vi "Teleop.vi"(10 "Match Info":T1={"Autonomous Elapsed Seconds"=0.0, "TeleOp Elapsed Seconds"=0.0, "Disabled Elapsed Seconds"=0.0, "Visited Autonomous"=FALSE, "Visited TeleOp"=FALSE, "Visited Disabled"=FALSE, "Autonomous Settings"={"Autonomous Style"=enum."Independent", "VI Refnum"=refnum}}, 11 "Call Context":T2) -> ()   [LabVIEW 2016]
doc: "This VI is called for each TeleOp packet received from the DS where the robot is not disabled. It is often used to read from the joysticks and update I/O or to update setpoints for timed control loops. It should complete and return within 20 milliseconds or it may miss DS packets."
uses:
  <vilib>/Rock Robotics/WPI/DriverStation/WPI_DriverStationDerivedRobotMode.ctl
  <vilib>/Rock Robotics/WPI/DriverStation/WPI_DriverStationMatch Info.ctl
  <vilib>/Rock Robotics/WPI/Solenoid/WPI_SolenoidValue.ctl
  <vilib>/Rock Robotics/WPI/ThirdParty/CanMotor/TalonSRX/WPI_CANTalonSRX_APIControlMode.ctl
  <vilib>/Rock Robotics/WPI/Utilities/WPI_GetSetVariantRefNum.vi
  <vilib>/Rock Robotics/Network Tables/NT Write Boolean Array.vi
  <vilib>/Rock Robotics/Network Tables/NT Write Numeric Array.vi
  <vilib>/Rock Robotics/Network Tables/NT Write Boolean.vi
  <vilib>/Rock Robotics/WPI/Solenoid/WPI_SolenoidSetEnum.vi
panel:
  out "Applied Throttle":dbl
  in  "Max Velocity":i32=63320
  in  "F":dbl
  in  "Speed PID":bool
  out "Setpoint vs Velocity":cluster{dbl, "Sensor Velocity":dbl}(graph)
  in  "Setpoint Control":bool
  out "Closed Loop Error":dbl(graph)
  in  "Setpoint (RPM)":dbl
  in  "D":dbl
  in  "I":dbl
  in  "P":dbl
  in  "Apply":bool
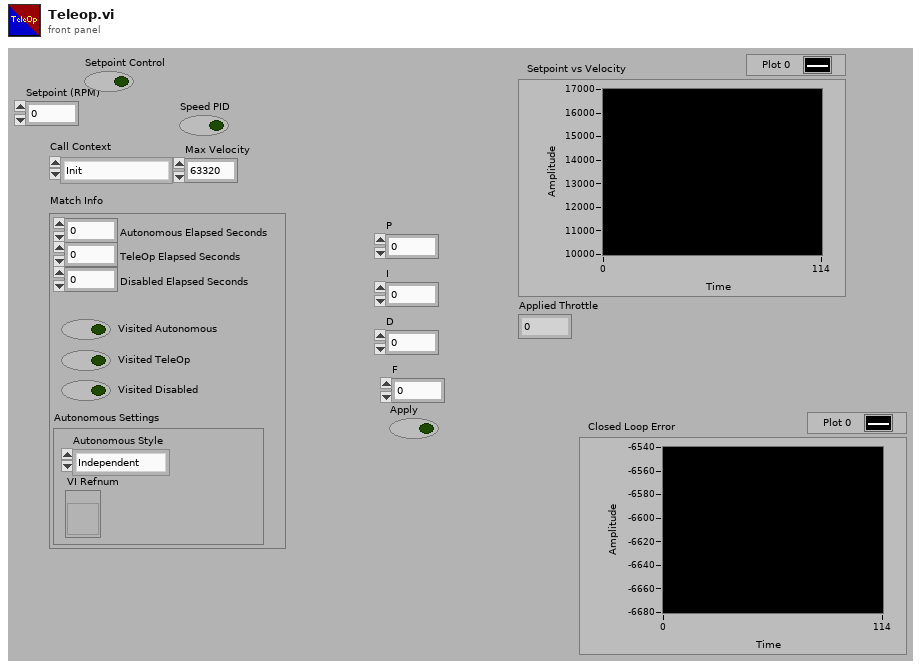
[diagram p1: front panel]
types:
  T1 = typedef "WPI_DriverStationMatch Info.ctl" = cluster{"Autonomous Elapsed Seconds":dbl, "TeleOp Elapsed Seconds":dbl, "Disabled Elapsed Seconds":dbl, "Visited Autonomous":bool, "Visited TeleOp":bool, "Visited Disabled":bool, "Autonomous Settings":cluster{"Autonomous Style":enum16{"Iterative", "Independent"}, "VI Refnum":refnum<vi>}}
  T2 = typedef "WPI_DriverStationDerivedRobotMode.ctl" = enum16{"Init", "Execute", "Stop"}
  T3 = typedef "WPI_JoystickDevRef.ctl" = cluster{"Device":T4}
  T4 = typedef "WPI_JoystickDeviceEnum.ctl" = enum16{"USB 0", "USB 1", "USB 2", "USB 3", "USB 4", "USB 5"}
  T5 = typedef "WPI_CANTalonSRX_APIControlMode.ctl" = enum8{"Percent VBus", "Speed", "Position", "Slave", "Unchanged / Invalid", "Voltage Compensation", "Current", "Motion Profile", "Motion Magic"}
  T6 = typedef "WPI_RobotDriveDevRef.ctl" = cluster{"DevStatus":errorcluster, "Motors[]":T7[], "Square Inputs":bool, "Max Output":dbl}
  T7 = typedef "WPI_MotorControlDeviceRef.ctl" = cluster{"DeviceStatus":errorcluster, "Type":T8, "PWM":cluster{"PWM Channel":T9, "DeadBand":T10}, "CAN":cluster{"Device Number":u8, "SetOutput VI Ref":variant, "GetOutput VI Ref":variant, "Enable VI Ref":variant, "Disable VI Ref":variant, "Data":variant}, "Invert":bool}
  T8 = typedef "WPI_MotorControlType.ctl" = enum16{"PWM", "CAN"}
  T9 = typedef "FPGA_DIOPWMChannel.ctl" = enum8{"PWM 0", "PWM 1", "PWM 2", "PWM 3", "PWM 4", "PWM 5", "PWM 6", "PWM 7", "PWM 8", "PWM 9", "PWM MXP 0", "PWM MXP 1", "PWM MXP 2", "PWM MXP 3", "PWM MXP 4", "PWM MXP 5", "PWM MXP 6", "PWM MXP 7", "PWM MXP 8", "PWM MXP 9", "Invalid"}
  T10 = typedef "WPI_PWMDeadband.ctl" = cluster{"Name":string, "maxPositivePwm":i32, "minPositivePwm":i32, "centerPwm":i32, "maxNegativePwm":i32, "minNegativePwm":i32, "angularRange":u16}
  T11 = typedef "WPI_CANTalonSRX_GlobalStatus.ctl" = cluster{"Applied Throttle":dbl, "Module Enabled":bool, "CAN Error":errorcluster, "Closed Loop Error":dbl, "Forward Limit Switch Closed":bool, "Reverse Limit Switch Closed":bool, "Sensor Position":dbl, "Sensor Velocity":dbl, "Current":dbl, "Sticky Fault - Over Temp":bool, "Sticky Fault - Under Voltage":bool, "Sticky Fault - Forward Limit":bool, "Sticky Fault - Reverse Limit":bool, "Sticky Fault - Forward Soft Limit":bool, "Sticky Fault - Reverse Soft Limit":bool, "Brake is Enabled":bool, "Encoder Position":dbl, "Encoder Velocity":dbl, "Encoder Index Count":dbl, "Encoder A Pin State":bool, "Encoder B Pin State":bool, "Encoder Index Pin State":bool, "Analog In":dbl, "Analog In Velocity":dbl, "Temperature (C)":dbl, "Battery Voltage":dbl, "Control 5 Is Supported":bool, "Current Profile Slot Select":dbl, "Pos Div 8":bool, "Vel Div 4":bool, "Pulse Width Position":i32, "Pulse Width Velocity":i32, "Pulse Width Rise To Rise (us)":i32, "Pulse Width Rise To Fall (us)":i32, "Mot Prof Active Is Under Run":bool, "Mot Prof Active Has Under Run":bool, "Mot Prof Active Is Last":bool, "Mot Prof Active Velocity Only":bool, "Mot Prof Active Is Valid":bool, "Mot Prof Buffer Is Full":bool, "Mot Prof Active Profile Slot Select":i32, "Mot Prof NextID":i32, "Mot Prof Count":i32, "Mot Prof Active Velocity":dbl, "Mot Prof Active Position":dbl, "Mot Prof Output Enable":i32}
  T12 = typedef "WPI_SolenoidValue.ctl" = enum16{"Off", "On", "Forward", "Reverse"}
  T13 = typedef "WPI_SolenoidDevRef.ctl" = cluster{"DevStatus":errorcluster, "Pneumatics Control Module":u8, "Forward Solenoid Channel":T14, "Reverse Solenoid Channel":T14}
  T14 = typedef "WPI_SolenoidChannel.ctl" = enum8{"Solenoid 0", "Solenoid 1", "Solenoid 2", "Solenoid 3", "Solenoid 4", "Solenoid 5", "Solenoid 6", "Solenoid 7", "Invalid"}
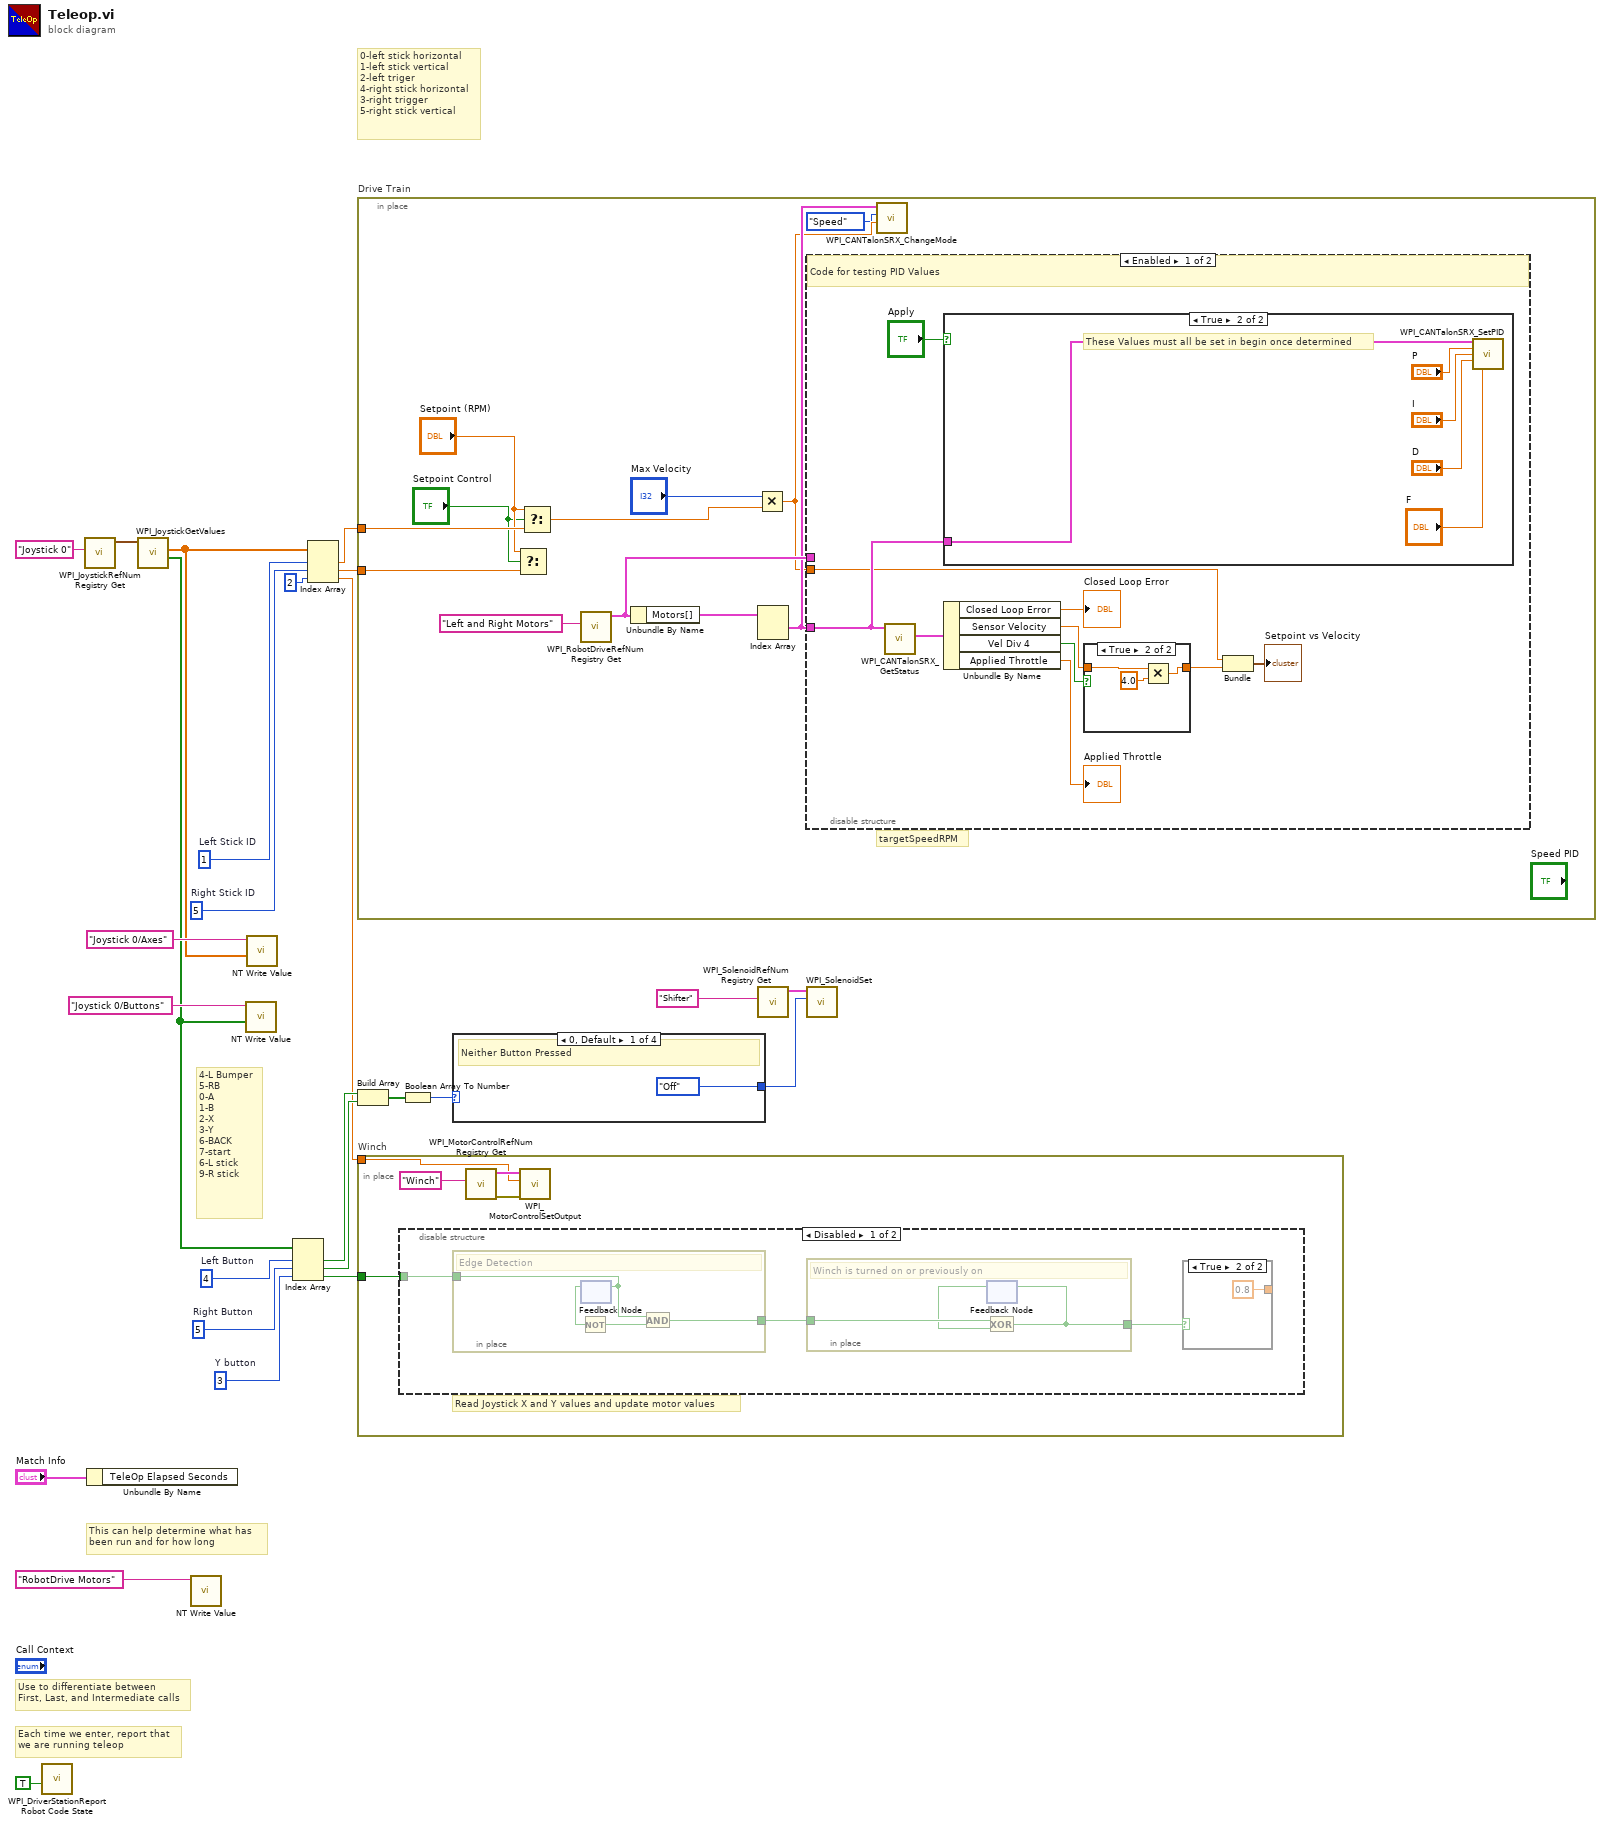
[diagram p0: block diagram]
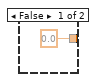
[diagram p5: hidden frame]
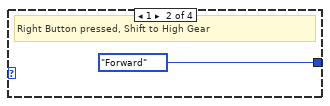
[diagram p7: hidden frame]
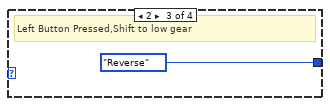
[diagram p8: hidden frame]
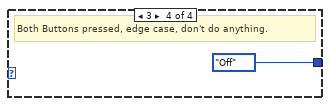
[diagram p9: hidden frame]
diagram:
  w4 = 3  # Y button
  w8 = 1  # Left Stick ID
  w7 = 5  # Right Stick ID
  w9 = 5  # Right Button
  w10 = 4  # Left Button
  # "0-left stick horizontal\n1-left stick vertical\n2-left triger\n4-right stick horizontal\n3-right trigger\n5-right stick vertical"
  # "4-L Bumper\n5-RB\n0-A\n1-B\n2-X\n3-Y\n6-BACK\n7-start\n6-L stick\n9-R stick"
  # "Each time we enter, report that\nwe are running teleop"
  # "Use to differentiate between\nFirst, Last, and Intermediate calls"
  # "This can help determine what has\nbeen run and for how long"
  n1 = call <vilib>:"WPI_DriverStationReport Robot Code State.vi"("TeleOp"=TRUE ("Autonomous")) -> ()  [unwired: 10 in, 1 out]
  n2 = call <vilib>:"WPI_JoystickRefNum Registry Get.vi"("refnum name"="Joystick 0") -> ("JoystickDevRef"=w24:T3)  [unwired: 1 in, 9 out]
  n3 = Unbundle By Name("Match Info") -> ()  [unwired: 1 out]
  n4 = call <vilib>:"WPI_JoystickGetValues.vi"("JoystickDevRef"=w24) -> ("Buttons"=w16:bool[], "Axes"=w20:dbl[])  [unwired: 6 in, 3 out]
  n5 = call-poly <vilib>:"NT Write Value.vi"("Name"="RobotDrive Motors") -> ()  [unwired: 10 in, 1 out]
  n6 = call-poly <vilib>:"NT Write Value.vi"("Boolean Array"=w16, "Name"="Joystick 0/Buttons") -> ()  [unwired: 9 in, 1 out]
  n7 = call-poly <vilib>:"NT Write Value.vi"("Numeric Array"=w20, "Name"="Joystick 0/Axes") -> ()  [unwired: 9 in, 1 out]
  n8 = Index Array(array=w16, index #1=w10, index #2=w9, index #3=w4) -> (element #1=w15:bool, element #2=w14:bool, element #3=w3:bool)
  n9 = Index Array(array=w20, index #1=w8, index #2=w7, index #3=2 ("index")) -> (element #1=w5:dbl, element #2=w6:dbl, element #3=w1:dbl)
  n10 = in-place "Drive Train" {
    in-place-border: w6 -> [w35]
    in-place-border: w5 -> [w37]
    # "targetSpeedRPM"
    n11 = Select(t="Setpoint (RPM)", s="Setpoint Control", f=w35) -> ()  [unwired: 1 out]
    n12 = Select(t="Setpoint (RPM)", s="Setpoint Control", f=w37) -> (s? t:f=w30:dbl)
    n13 = call <vilib>:"WPI_RobotDriveRefNum Registry Get.vi"("refnum name"="Left and Right Motors") -> ("RobotDriveDevRef"=w32:T6)  [unwired: 1 in, 9 out]
    n14 = Unbundle By Name(w32) -> ("Motors[]"=w33:T7[])
    n15 = Multiply(x="Max Velocity", y=w30) -> (x*y=w28:dbl)
    n16 = Index Array(array=w33) -> (element #1=w31:T7)  [unwired: 2 in, 1 out]
    n17 = disable-structure shown="Enabled" {
      disable-tunnel: w32 -> [_ _]
      disable-tunnel: w31 -> [w41 _]
      disable-tunnel: w28 -> [w40 _]
      frame Enabled {
        # "Code for testing PID Values"
        n18 = call <vilib>:"WPI_CANTalonSRX_GetStatus.vi"("CAN Talon SRX Ref"=w41) -> ("Talon SRX Status"=w48:T11)  [unwired: 8 in, 2 out]
        n19 = case shown="True" "Apply" {
          tunnel: w41 -> [_ w53]
          frame False {
          }
          frame True {
            # "These Values must all be set in begin once determined"
            n20 = call <vilib>:"WPI_CANTalonSRX_SetPID.vi"("CAN Talon SRX Ref"=w53, "P"="P", "I"="I", "D"="D", "F"="F") -> ()  [unwired: 9 in, 2 out]
          }
        }
        n21 = Unbundle By Name(w48) -> ("Closed Loop Error"=→"Closed Loop Error":dbl, "Sensor Velocity"=w42:dbl, "Vel Div 4"=w44:bool, "Applied Throttle"=→"Applied Throttle":dbl)
        n22 = case shown="True" w44 {
          tunnel: [w49 w52] -> w43
          tunnel: w42 -> [w49 w51]
          frame False {
          }
          frame True {
            n23 = Multiply(x=w51, y=4.0) -> (x*y=w52:dbl)
          }
        }
        n24 = Bundle(w40, "Sensor Velocity"=w43) -> (→"Setpoint vs Velocity":cluster{dbl, "Sensor Velocity":dbl})  [unwired: 1 in]
      }
      frame Disabled {
      }
    }
    n25 = call <vilib>:"WPI_CANTalonSRX_ChangeMode.vi"("Output"=w28, "Control Mode"=WPI_CANTalonSRX_APIControlMode."Speed", "CAN Talon SRX Ref"=w31) -> ()  [unwired: 7 in, 2 out]
  }
  n26 = Build Array(w15, w14) -> (w13:bool[])
  n27 = in-place "Winch" {
    in-place-border: w3 -> [w59]
    in-place-border: w1 -> [w58]
    # "Read Joystick X and Y values and update motor values"
    n28 = disable-structure shown="Disabled" {
      disable-tunnel: w59 -> [w65 _]
      frame Disabled {
        n29 = in-place {
          in-place-border: w65 -> [w74]
          in-place-border: [w71] -> w64
          # "Edge Detection"
          n30 = feedback #1() -> (w72:bool)  [unwired: 1 in]
          n31 = Not(x=w72) -> (.not. x?=w73:bool)
          n32 = feedback-in #1(w74) -> ()
          n33 = And(x=w74, y=w73) -> (x .and. y?=w71:bool)
        }
        n34 = in-place {
          in-place-border: w64 -> [w68]
          in-place-border: [w67] -> w63
          # "Winch is turned on or previously on"
          n35 = feedback #2() -> (w66:bool)  [unwired: 1 in]
          n36 = Exclusive Or(1:w66, 2:w68) -> (0:w67:bool)
          n37 = feedback-in #2(w67) -> ()
        }
        n38 = case shown="True" w63 {
          tunnel: [0.0 ("Output") 0.8 ("Output")] -> _
          frame False {
          }
          frame True {
          }
        }
      }
      frame Enabled {
      }
    }
    n39 = call <vilib>:"WPI_MotorControlRefNum Registry Get.vi"("refnum name"="Winch") -> ("error out"=w61:errorcluster, "MotorControlDevRef"=w60:T7)  [unwired: 9 in]
    n40 = call <vilib>:"WPI_MotorControlSetOutput.vi"("error in (no error)"=w61, "Output"=w58, "MotorControlDevRef"=w60) -> ()  [unwired: 6 in, 3 out]
  }
  n41 = Boolean Array To Number(Boolean array=w13) -> (number=w12:u32)
  n42 = case shown="0, Default" w12 {
    tunnel: [WPI_SolenoidValue."Off" ("Value") WPI_SolenoidValue."Forward" ("Value") WPI_SolenoidValue."Reverse" ("Value") WPI_SolenoidValue."Off" ("Value")] -> w11
    frame 0, Default {
      # "Neither Button Pressed"
    }
    frame 1 {
      # "Right Button pressed, Shift to High Gear"
    }
    frame 2 {
      # "Left Button Pressed,Shift to low gear"
    }
    frame 3 {
      # "Both Buttons pressed, edge case, don't do anything."
    }
  }
  n43 = call <vilib>:"WPI_SolenoidRefNum Registry Get.vi"("refnum name"="Shifter") -> ("SolenoidDevRef"=w17:T13)  [unwired: 9 in, 1 out]
  n44 = call-poly <vilib>:"WPI_SolenoidSet.vi"("Value"=w11, "SolenoidDevRef"=w17) -> ()  [unwired: 8 in, 2 out]
